vi "按鈕Tool Initial.vi"() -> (0 "error IO":errorcluster)   [LabVIEW 2019]
uses:
  Global/Process Global.vi
panel:
  in  "$Read Project Recipe":path=path "C:/Users/MyUser/Desktop/S2_Project.txt"
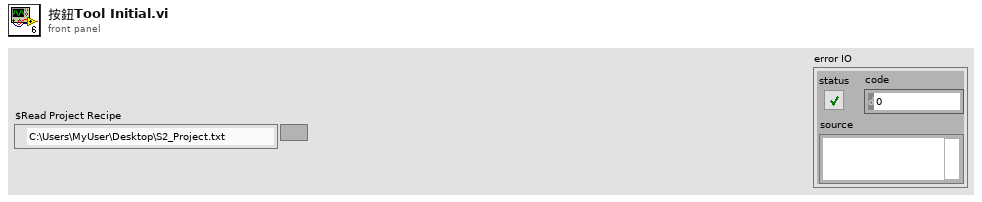
[diagram p1: front panel]
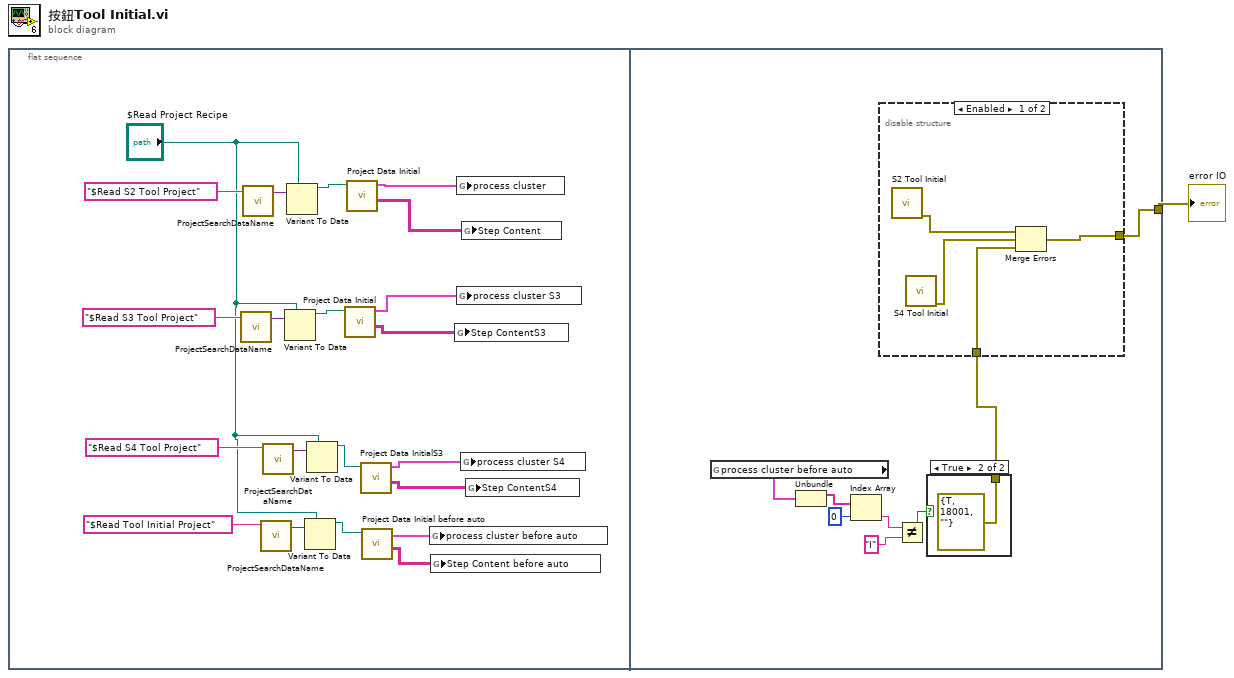
[diagram p0: block diagram]
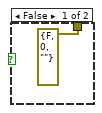
[diagram p2: hidden frame]
diagram:
  n1 = flat-sequence {
    tunnel: [w30] -> w1
    frame #0 {
      n2 = call "ProjectSearchDataName.vi"("element"="$Read S3 Tool Project") -> ("variant"=w11:variant)  [unwired: 7 in, 3 out]
      n3 = call "ProjectSearchDataName.vi"("element"="$Read S2 Tool Project") -> ("variant"=w16:variant)  [unwired: 7 in, 3 out]
      n4 = call "ProjectSearchDataName.vi"("element"="$Read Tool Initial Project") -> ("variant"=w4:variant)  [unwired: 7 in, 3 out]
      n5 = call "ProjectSearchDataName.vi"("element"="$Read S4 Tool Project") -> ("variant"=w8:variant)  [unwired: 7 in, 3 out]
      n6 = Variant To Data(type="$Read Project Recipe", Variant=w11) -> (data=w13:path)  [unwired: 1 in, 1 out]
      n7 = Variant To Data(type="$Read Project Recipe", Variant=w16) -> (data=w14:path)  [unwired: 1 in, 1 out]
      n8 = Variant To Data(type="$Read Project Recipe", Variant=w4) -> (data=w3:path)  [unwired: 1 in, 1 out]
      n9 = Variant To Data(type="$Read Project Recipe", Variant=w8) -> (data=w6:path)  [unwired: 1 in, 1 out]
      n10 = call "Project Data Initial.vi"("configuration file path"=w13) -> ("Step Content"=w10:string[][], "process cluster"=w9:cluster{string[], i32[]})  [unwired: 7 in, 2 out]
      n11 = call "Project Data Initial.vi"("configuration file path"=w14) -> ("Step Content"=w21:string[][], "process cluster"=w22:cluster{string[], i32[]})  [unwired: 7 in, 2 out]
      n12 = call "Project Data InitialS3.vi"("configuration file path"=w6) -> ("Step Content"=w20:string[][], "process cluster"=w19:cluster{string[], i32[]})  [unwired: 8 in, 1 out]
      n13 = call "Project Data Initial before auto.vi"("configuration file path"=w3) -> ("Step Content"=w17:string[][], "process cluster"=w18:cluster{string[], i32[]})  [unwired: 7 in, 2 out]
      n14 = global write "Process Global.vi" "process cluster before auto"(w18) -> ()
      n15 = global write "Process Global.vi" "Step Content before auto"(w17) -> ()
      n16 = global write "Process Global.vi" "Step ContentS3"(w10) -> ()
      n17 = global write "Process Global.vi" "process cluster"(w22) -> ()
      n18 = global write "Process Global.vi" "process cluster S3"(w9) -> ()
      n19 = global write "Process Global.vi" "process cluster S4"(w19) -> ()
      n20 = global write "Process Global.vi" "Step Content"(w21) -> ()
      n21 = global write "Process Global.vi" "Step ContentS4"(w20) -> ()
    }
    frame #1 {
      n22 = global read "Process Global.vi" "process cluster before auto"() -> (w29:cluster{string[], i32[]})
      n23 = Unbundle(w29) -> (w28:string[])  [unwired: 1 out]
      n24 = Index Array(array=w28, index=0) -> (element=w25:string)
      n25 = Not Equal?(x=w25, y="I") -> (x != y?=w23:bool)
      n26 = case shown="True" w23 {
        tunnel: [errorcluster {"status"=FALSE, "code"=0, "source"=""} ("error constant") errorcluster {"status"=TRUE, "code"=18001, "source"=""} ("error constant")] -> w24
        frame False {
        }
        frame True {
        }
      }
      n27 = disable-structure shown="Enabled" {
        disable-tunnel: [w34 _] -> w30
        disable-tunnel: w24 -> [w33 _]
        frame Enabled {
          n28 = call "S2 Tool Initial.vi"() -> ("error constant"=w36:errorcluster)  [unwired: 10 in, 1 out]
          n29 = call "S4 Tool Initial.vi"() -> ("error constant"=w35:errorcluster)  [unwired: 10 in, 1 out]
          n30 = Merge Errors(w36, w35, w33) -> (w34:errorcluster)
        }
        frame Disabled {
        }
      }
    }
  }
  "error IO" <- w1
